vi "MB_Master Comm Tester.vi"() -> ()   [LabVIEW 2012]
doc: "Modbus Comm Tester\n\nThis VI demonstrates the usage of the Modbus Master API for both TCP and Serial connections.\nIt is also a useful tool for testing communication with your modbus device. You can test different\ncommunication parameters and coil/register address ranges without having to write any code.\n\nCopyright (c) 2016, Plasmionique Inc.\nAll rights reserved.\n\nLicense: BSD (2-Clause) - http://opensource.org/licenses/BSD-2-Clause"
uses:
  MB_Master/MB_Master.lvclass
  MB_Master_TCP/MB_Master_TCP.lvclass
  MB_ADU/MB_ADU.lvclass/MB_ADU.ctl
  MB_ADU/Read TX Data.vi
  MB_ADU/Read RX Data.vi
  MB_ADU/Read RX Timestamp.vi
  MB_Master_Serial/MB_Master_Serial.lvclass
  MB Master.lvlib
  MB_ADU/MB_ADU.lvclass
panel:
  in  "Poll Period (ms)":i32=100
  in  "Tab Control":enum32{"Page 1", "Page 2"}(tab)
  in  "Retries":i32=1
  in  "Timeout (ms)":u32=300
  in  "Flow Control":u16(ring) items=["None", "XON/XOFF", "RTS/CTS", "XON/XOFF & RTS/CTS", "DTR/DSR", "XON/XOFF & DTR/DSR"]
  in  "Parity":u16(ring) items=["None", "Odd", "Even", "Mark", "Space"]
  in  "Stop Bits":u16(ring)=10 items=["1.0"=10, "1.5"=15, "2.0"=20]
  in  "Baud Rate (bps)":u32(ring)=19200 items=["9600"=9600, "19200"=19200, "38400"=38400, "57600"=57600, "115200"=115200, "460800"=460800, "921600"=921600]
  in  "Slave Address":u8=1
  in  "Mode":enum16{"RTU", "ASCII"}(ring)
  in  "COM Port":refnum<visa-resource-name>
  in  "TCP_Port":u16=502 caption="Port"
  in  "IP Address":string="localhost"
  in  "TCP_Timeout":i32=10000 caption="Timeout (ms)"
  in  "TCP_Slave ID":u8=255 caption="Slave ID" format="%.0x"
  in  "Type":enum16{"Serial", "TCP"}(ring) caption="Connection Type"
  out "dt (ms)":u32
  in  "DI Poll":bool
  in  "IR Poll":bool
  in  "Exit":bool
  out "Last Error Time":string
  out "Last RX Time":string
  in  "Write Hld Regs":bool
  in  "Read Hld Regs":bool
  in  "HR QTY":u16=1 caption="Quantity"
  in  "HR SA":u16 caption="Starting Address" format="%.0x"
  in  "Holding Registers":u16[](array[numeric])
  in  "Read In Regs":bool
  in  "IR QTY":u16=1 caption="Quantity"
  in  "IR SA":u16 caption="Starting Address" format="%.0x"
  out "Input Registers":u16[](array[numeric])
  in  "Read DIs":bool
  in  "DI QTY":u16=1 caption="Quantity"
  in  "DI SA":u16 caption="Starting Address" format="%.0x"
  out "Discrete Inputs":bool[](array[boolean])
  in  "Write Coils":bool
  in  "Read Coils":bool
  in  "Coil QTY":u16=1 caption="Quantity"
  in  "Coil SA":u16 caption="Starting Address" format="%.0x"
  in  "Coils":bool[](array[boolean])
  out "Last TX":string
  out "Last RX":string
  out "Last Error Status":errorcluster
  out "Open?":bool
  in  "Close":bool
  in  "Open":bool
  # "Input Registers"
  # "Discrete Inputs"
  # "Communication Settngs"
  # "Communication Status"
  # "Holding Registers"
  # "Coils"
  # "See block diagram for description and usage notes."
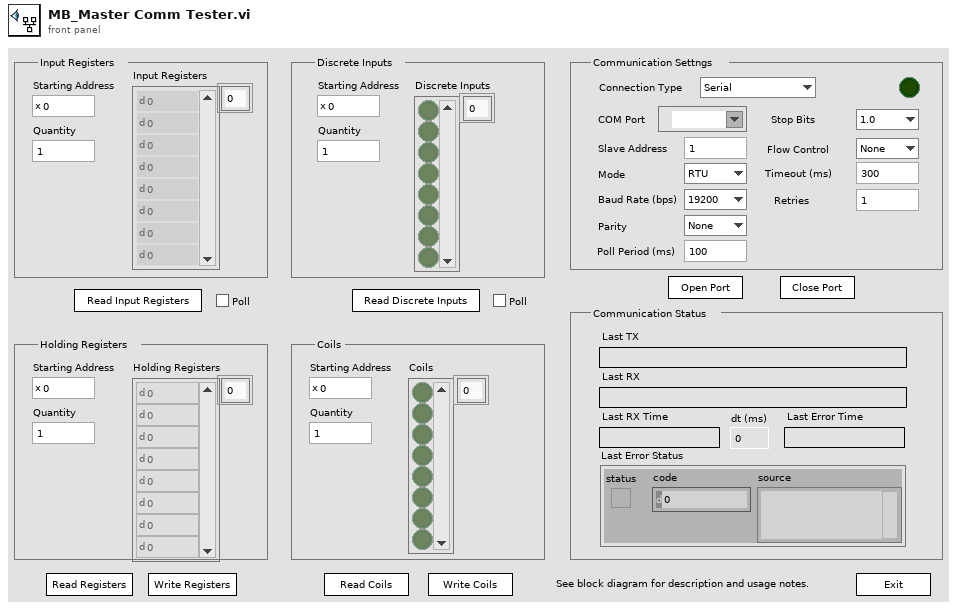
[diagram p1: front panel]
types:
  T1 = cluster{"baud rate (bps)":u32, "stop bits":u16, "parity":u16, "flow control":u16, "timeout":u32, "retries":i32}
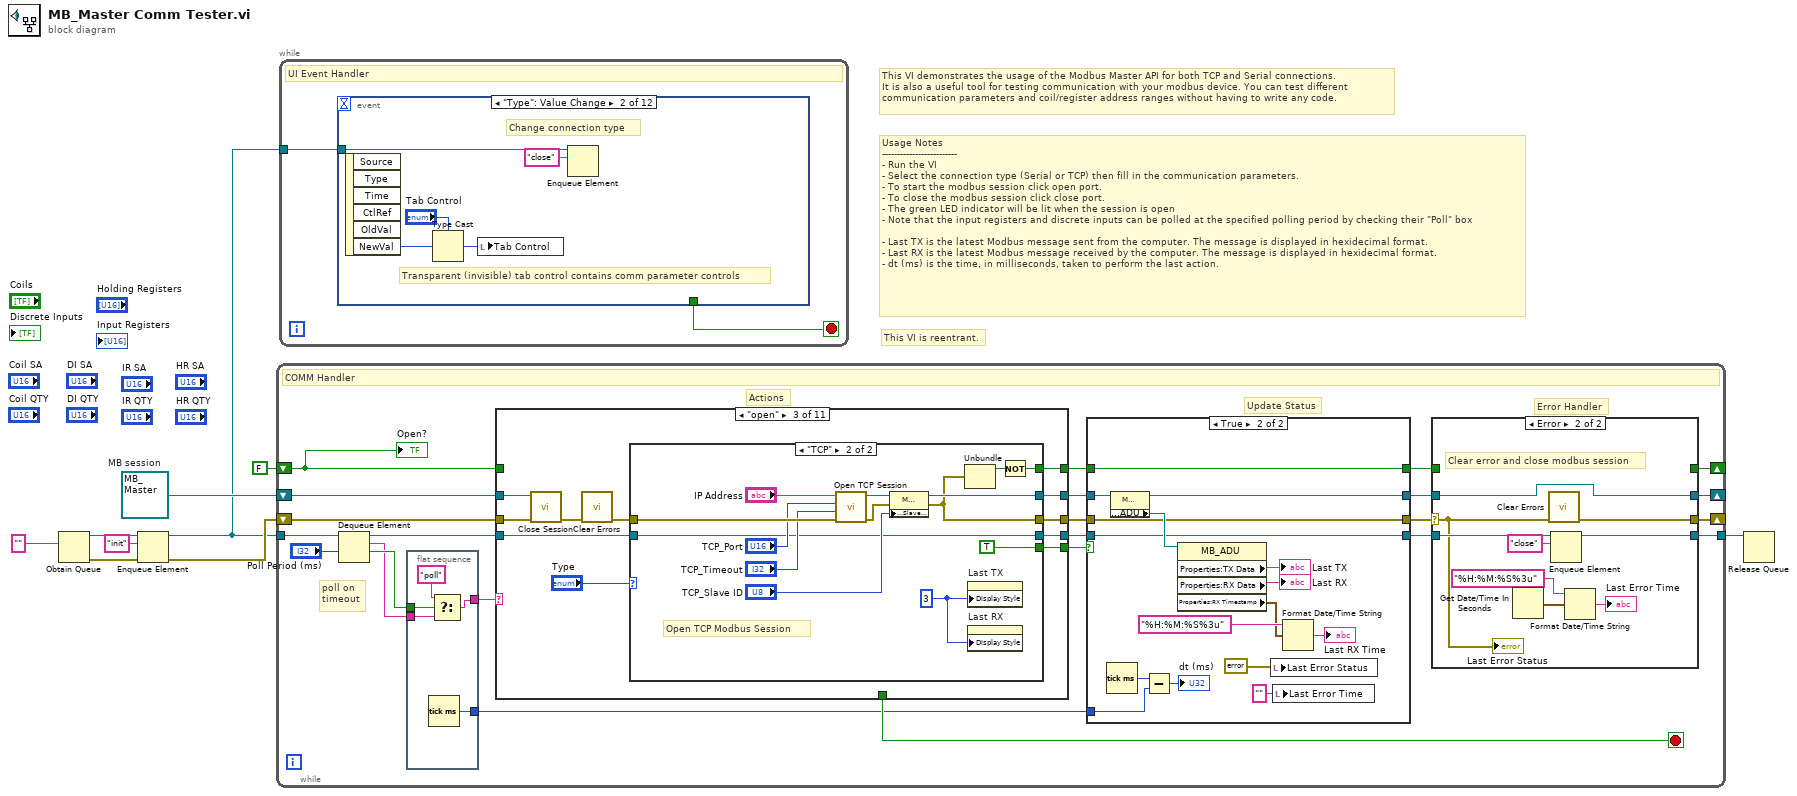
[diagram p0: block diagram]
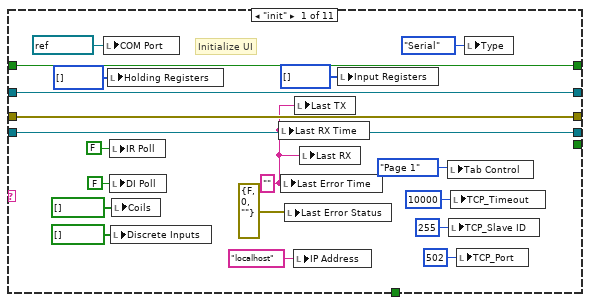
[diagram p4: hidden frame]
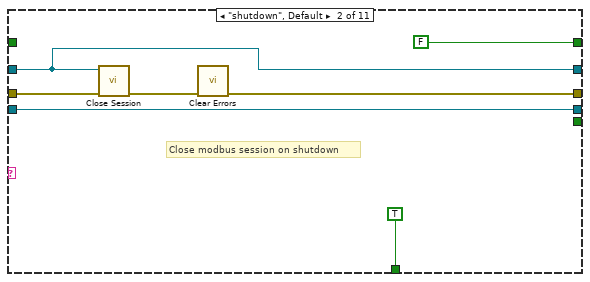
[diagram p5: hidden frame]
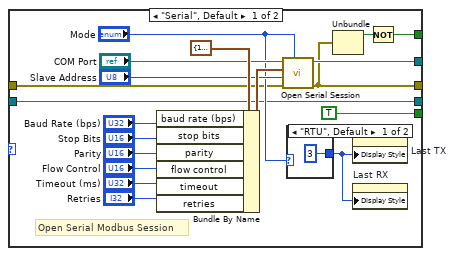
[diagram p6: hidden frame]
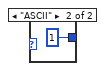
[diagram p7: hidden frame]
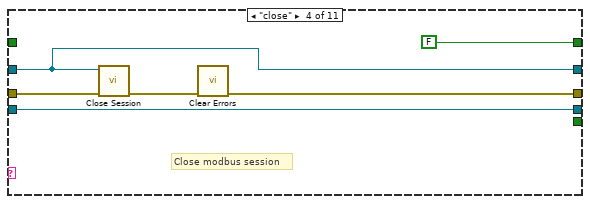
[diagram p8: hidden frame]
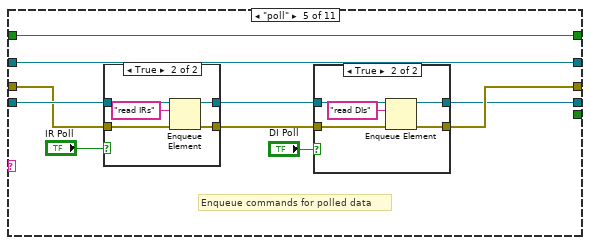
[diagram p9: hidden frame]
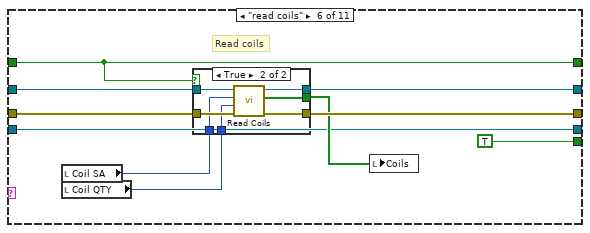
[diagram p12: hidden frame]
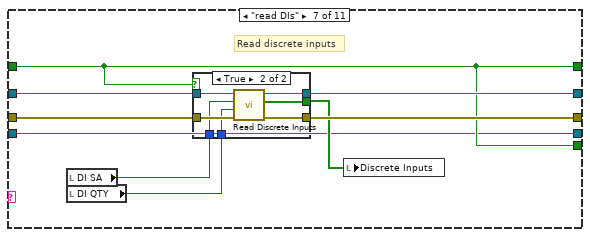
[diagram p14: hidden frame]
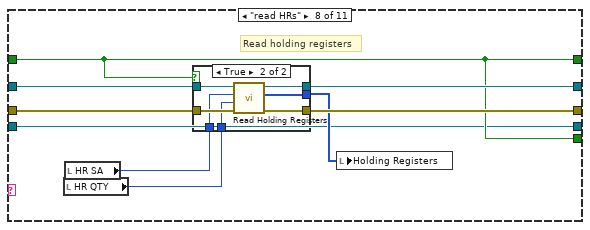
[diagram p16: hidden frame]
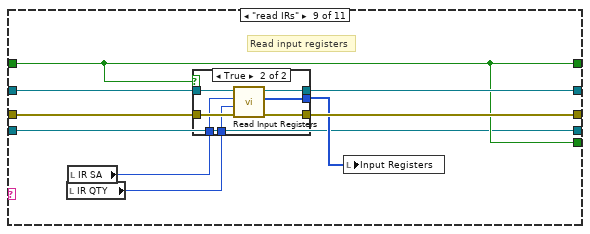
[diagram p18: hidden frame]
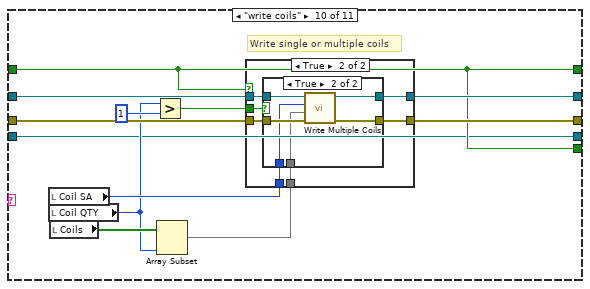
[diagram p20: hidden frame]
diagram:
  w7 = refnum<class "MB_Master.lvclass"> refnum  # MB session
  # "This VI is reentrant."
  # "Usage Notes\n-------------------------\n- Run the VI\n- Select the connection type (Serial or TCP) then fill in the communication parameters.\n- To start the modbus session click open port.\n- To close the modbus session click close port.\n- The green LED indicator will be lit when the session is open\n- Note that the input registers and discrete inputs can be polled at the specified polling period by checking their \"Poll\" box\n\n- Last TX is the latest Modbus message sent from the computer. The message is displayed in hexidecimal format.\n- Last RX is the latest Modbus message received by the computer. The message is displayed in hexidecimal format. \n- dt (ms) is the time, in milliseconds, taken to perform the last action."
  # "This VI demonstrates the usage of the Modbus Master API for both TCP and Serial connections.\nIt is also a useful tool for testing communication with your modbus device. You can test different\ncommunication parameters and coil/register address ranges without having to write any code."
  n1 = Obtain Queue(element data type="") -> (queue out=w6:refnum<queue>, error out=w4:errorcluster)  [unwired: 4 in, 1 out]
  n2 = Enqueue Element(queue=w6, element="init", error in (no error)=w4) -> (queue out=w2:refnum<queue>, error out=w3:errorcluster)  [unwired: 1 in, 1 out]
  n3 = while {
    tunnel: w2 -> [w33]
    shift-right: [w16] -> _
    shift-left: w7 -> [w32]
    shift-right: [w23] -> _
    shift-left: w3 -> [w24]
    shift-right: [w18] -> _
    shift-left: FALSE -> [w28]
    tunnel: [w22] -> w1
    stop <- w31 stop-if-true
    # "poll on\ntimeout"
    # "Actions"
    # "Error Handler"
    # "Update Status"
    # "COMM Handler"
    n4 = Dequeue Element(queue=w33, timeout in ms (-1)="Poll Period (ms)") -> (queue out=w30:refnum<queue>, element=w20:string, timed out?=w21:bool)  [unwired: 1 in, 1 out]
    n5 = flat-sequence {
      tunnel: [w51] -> w25
      tunnel: w21 -> [w50]
      tunnel: w20 -> [w49]
      tunnel: [w47] -> w19
      frame #0 {
        n6 = Tick Count (ms)() -> (millisecond timer value=w51:u32)
        n7 = Select(t="poll", s=w50, f=w49) -> (s? t:f=w47:string)
      }
    }
    n8 = case shown="\"open\"" w19 {
      tunnel: [w89 w94 w108 w146 w151 w181 w199 w217 w235 w255 w289] -> w29
      tunnel: w32 -> [w89 w94 w103 w146 w151 w183 w201 w219 w237 w258 w292]
      tunnel: [w88 w95 w107 w147 w153 w180 w198 w216 w234 w253 w287] -> w13
      tunnel: w24 -> [w88 w97 w102 w149 w156 w182 w200 w218 w236 w254 w288]
      tunnel: [_ TRUE _ _ _ _ _ _ _ _ _] -> w31
      tunnel: w30 -> [w79 w91 w99 w144 w158 w174 w193 w211 w229 w247 w281]
      tunnel: w28 -> [w86 _ _ _ w152 w178 w194 w212 w230 w248 w282]
      tunnel: [w86 FALSE w106 FALSE w152 w178 w194 w212 w230 w248 w282] -> w15
      tunnel: [_ _ w105 _ _ TRUE w194 w212 w230 w248 w282] -> w27
      tunnel: [w79 w91 w98 w144 w150 w174 w193 w211 w229 w247 w281] -> w11
      frame "init" {
        w87 = "" ("Last Error Time")
        # "Initialize UI"
        n9 = local write "COM Port"(refnum<visa-resource-name> refnum ("COM Port")) -> ()
        n10 = local write "Holding Registers"(u16[] [] ("Holding Registers")) -> ()
        n11 = local write "IR Poll"(FALSE ("IR Poll")) -> ()
        n12 = local write "DI Poll"(FALSE ("DI Poll")) -> ()
        n13 = local write "Discrete Inputs"(bool[] [] ("Coils")) -> ()
        n14 = local write "Coils"(bool[] [] ("Coils")) -> ()
        n15 = local write "Last RX Time"(w87) -> ()
        n16 = local write "Last Error Time"(w87) -> ()
        n17 = local write "Last Error Status"(errorcluster {"status"=FALSE, "code"=0, "source"=""} ("Last Error Status")) -> ()
        n18 = local write "IP Address"("localhost" ("IP Address")) -> ()
        n19 = local write "Last TX"(w87) -> ()
        n20 = local write "Last RX"(w87) -> ()
        n21 = local write "Input Registers"(u16[] [] ("Input Registers")) -> ()
        n22 = local write "Tab Control"(enum32{"Page 1", "Page 2"}."Page 1" ("Tab Control")) -> ()
        n23 = local write "TCP_Slave ID"(u8 255 ("TCP_Slave ID")) -> ()
        n24 = local write "TCP_Timeout"(10000 ("TCP_Timeout")) -> ()
        n25 = local write "TCP_Port"(u16 502 ("TCP_Port")) -> ()
        n26 = local write "Type"(enum16{"Serial", "TCP"}."Serial" ("Type")) -> ()
      }
      frame "shutdown", Default {
        # "Close modbus session on shutdown"
        n27 = call-dynamic "Close Session.vi"("error in (no error)"=w97, "MB session in"=w94) -> ("error out"=w96:errorcluster)  [unwired: 9 in]
        n28 = call <vilib>:"Clear Errors.vi"("error in (no error)"=w96) -> ("error out"=w95:errorcluster)  [unwired: 6 in]
      }
      frame "open" {
        n29 = call-dynamic "Close Session.vi"("error in (no error)"=w102, "MB session in"=w103) -> ("error out"=w104:errorcluster)  [unwired: 9 in]
        n30 = call <vilib>:"Clear Errors.vi"("error in (no error)"=w104) -> ("error out"=w101:errorcluster)  [unwired: 6 in]
        n31 = case shown="\"TCP\"" "Type" {
          tunnel: [w117 w134] -> w108
          tunnel: [w116 w132] -> w107
          tunnel: [w114 w131] -> w106
          tunnel: [TRUE TRUE] -> w105
          tunnel: w101 -> [w110 w141]
          tunnel: [w109 w135] -> w98
          tunnel: w99 -> [w109 w135]
          frame "Serial", Default {
            # "Open Serial Modbus Session"
            n32 = Bundle By Name(cluster=T1 {"baud rate (bps)"=19200, "stop bits"=10, "parity"=0, "flow control"=0, "timeout"=1000, "retries"=1} ("Serial Config"), "baud rate (bps)"="Baud Rate (bps)", "stop bits"="Stop Bits", "parity"="Parity", "flow control"="Flow Control", "timeout"="Timeout (ms)", "retries"="Retries") -> (w119:T1)
            n33 = call "Open Serial Session.vi"("Mode (RTU)"="Mode", "Error in"=w110, "Slave ID"="Slave Address", "Serial Config"=w119, "VISA Resource"="COM Port") -> ("Error out"=w116:errorcluster, "MB_Serial session"=w117:refnum<class "MB_Master_Serial.lvclass">)  [unwired: 5 in]
            n34 = case shown="\"RTU\", Default" "Mode" {
              tunnel: [u32 3 ("Display Style") u32 1 ("Display Style")] -> w111
              frame "RTU", Default {
              }
              frame "ASCII" {
              }
            }
            n35 = Unbundle(w116) -> ("status"=w115:bool)  [unwired: 2 out]
            n36 = property on="Last TX" class="Str"("Display Style"=w111) -> ()  [unwired: 2 in, 2 out]
            n37 = property on="Last RX" class="Str"("Display Style"=w111) -> ()  [unwired: 2 in, 2 out]
            n38 = Not(x=w115) -> (.not. x?=w114:bool)
          }
          frame "TCP" {
            w130 = u32 3 ("Display Style")
            # "Open TCP Modbus Session"
            n39 = call "Open TCP Session.vi"("error in (no error)"=w141, "Timeout (10000)"="TCP_Timeout", "Port (502)"="TCP_Port", "IP Address"="IP Address") -> ("error out"=w142:errorcluster, "MB_TCP session"=w143:refnum<class "MB_Master_TCP.lvclass">)  [unwired: 6 in]
            n40 = property class="MB_Master_TCP"(reference=w143, error in=w142, "Properties:Slave ID"="TCP_Slave ID") -> (reference out=w134:refnum<class "MB_Master_TCP.lvclass">, error out=w132:errorcluster)
            n41 = Unbundle(w132) -> ("status"=w133:bool)  [unwired: 2 out]
            n42 = property on="Last TX" class="Str"("Display Style"=w130) -> ()  [unwired: 2 in, 2 out]
            n43 = property on="Last RX" class="Str"("Display Style"=w130) -> ()  [unwired: 2 in, 2 out]
            n44 = Not(x=w133) -> (.not. x?=w131:bool)
          }
        }
      }
      frame "close" {
        # "Close modbus session"
        n45 = call-dynamic "Close Session.vi"("error in (no error)"=w149, "MB session in"=w146) -> ("error out"=w148:errorcluster)  [unwired: 9 in]
        n46 = call <vilib>:"Clear Errors.vi"("error in (no error)"=w148) -> ("error out"=w147:errorcluster)  [unwired: 6 in]
      }
      frame "poll" {
        # "Enqueue commands for polled data"
        n47 = case shown="True" "IR Poll" {
          tunnel: w158 -> [w168 w172]
          tunnel: [w168 w171] -> w157
          tunnel: w156 -> [w167 w170]
          tunnel: [w167 w169] -> w154
          frame False {
          }
          frame True {
            n48 = Enqueue Element(queue=w172, element="read IRs", error in (no error)=w170) -> (queue out=w171:refnum<queue>, error out=w169:errorcluster)  [unwired: 1 in, 1 out]
          }
        }
        n49 = case shown="True" "DI Poll" {
          tunnel: w157 -> [w160 w165]
          tunnel: w154 -> [w161 w164]
          tunnel: [w161 w163] -> w153
          tunnel: [w160 w162] -> w150
          frame False {
          }
          frame True {
            n50 = Enqueue Element(queue=w165, element="read DIs", error in (no error)=w164) -> (queue out=w162:refnum<queue>, error out=w163:errorcluster)  [unwired: 1 in, 1 out]
          }
        }
      }
      frame "read coils" {
        # "Read coils"
        n51 = local read "Coil SA"() -> (w177:u16)
        n52 = local read "Coil QTY"() -> (w176:u16)
        n53 = case shown="True" w178 {
          tunnel: w183 -> [w185 w192]
          tunnel: w182 -> [w184 w191]
          tunnel: [w185 w190] -> w181
          tunnel: [w184 w189] -> w180
          tunnel: w177 -> [_ w188]
          tunnel: w176 -> [_ w187]
          tunnel: [_ w186] -> w179
          frame False {
          }
          frame True {
            n54 = call "Read Coils.vi"("error in (no error)"=w191, "quantity"=w187, "starting address"=w188, "MB session in"=w192) -> ("error out"=w189:errorcluster, "Coils"=w186:bool[], "MB session out"=w190:refnum<class "MB_Master.lvclass">)  [unwired: 5 in]
          }
        }
        n55 = local write "Coils"(w179) -> ()
      }
      frame "read DIs" {
        # "Read discrete inputs"
        n56 = local read "DI SA"() -> (w196:u16)
        n57 = local read "DI QTY"() -> (w195:u16)
        n58 = case shown="True" w194 {
          tunnel: w201 -> [w203 w210]
          tunnel: w200 -> [w202 w209]
          tunnel: [w203 w208] -> w199
          tunnel: [w202 w207] -> w198
          tunnel: w196 -> [_ w206]
          tunnel: w195 -> [_ w205]
          tunnel: [_ w204] -> w197
          frame False {
          }
          frame True {
            n59 = call "Read Discrete Inputs.vi"("error in (no error)"=w209, "quantity"=w205, "starting address"=w206, "MB session in"=w210) -> ("error out"=w207:errorcluster, "Inputs"=w204:bool[], "MB session out"=w208:refnum<class "MB_Master.lvclass">)  [unwired: 5 in]
          }
        }
        n60 = local write "Discrete Inputs"(w197) -> ()
      }
      frame "read HRs" {
        # "Read holding registers"
        n61 = local read "HR QTY"() -> (w213:u16)
        n62 = local read "HR SA"() -> (w214:u16)
        n63 = case shown="True" w212 {
          tunnel: w219 -> [w221 w228]
          tunnel: w218 -> [w220 w227]
          tunnel: [w221 w226] -> w217
          tunnel: [w220 w225] -> w216
          tunnel: w214 -> [_ w224]
          tunnel: w213 -> [_ w223]
          tunnel: [_ w222] -> w215
          frame False {
          }
          frame True {
            n64 = call "Read Holding Registers.vi"("error in (no error)"=w227, "quantity"=w223, "starting address"=w224, "MB session in"=w228) -> ("error out"=w225:errorcluster, "Registers"=w222:u16[], "MB session out"=w226:refnum<class "MB_Master.lvclass">)  [unwired: 5 in]
          }
        }
        n65 = local write "Holding Registers"(w215) -> ()
      }
      frame "read IRs" {
        # "Read input registers"
        n66 = local read "IR QTY"() -> (w231:u16)
        n67 = local read "IR SA"() -> (w232:u16)
        n68 = case shown="True" w230 {
          tunnel: w237 -> [w239 w246]
          tunnel: w236 -> [w238 w245]
          tunnel: [w239 w244] -> w235
          tunnel: [w238 w243] -> w234
          tunnel: w232 -> [_ w242]
          tunnel: w231 -> [_ w241]
          tunnel: [_ w240] -> w233
          frame False {
          }
          frame True {
            n69 = call "Read Input Registers.vi"("error in (no error)"=w245, "quantity"=w241, "starting address"=w242, "MB session in"=w246) -> ("error out"=w243:errorcluster, "Registers"=w240:u16[], "MB session out"=w244:refnum<class "MB_Master.lvclass">)  [unwired: 5 in]
          }
        }
        n70 = local write "Input Registers"(w233) -> ()
      }
      frame "write coils" {
        # "Write single or multiple coils"
        n71 = local read "Coil SA"() -> (w252:u16)
        n72 = local read "Coil QTY"() -> (w250:u16)
        n73 = local read "Coils"() -> (w251:bool[])
        n74 = Greater?(x=w250, y=u16 1) -> (0:w256:bool)
        n75 = Array Subset(array=w251, length=w250) -> (w249:bool[])  [unwired: 1 in]
        n76 = case shown="True" w248 {
          tunnel: w258 -> [w260 w267]
          tunnel: w256 -> [_ w266]
          tunnel: [w260 w265] -> w255
          tunnel: w254 -> [w259 w264]
          tunnel: [w259 w263] -> w253
          tunnel: w252 -> [_ w262]
          tunnel: w249 -> [_ w261]
          frame False {
          }
          frame True {
            n77 = case shown="True" w266 {
              tunnel: w267 -> [w274 w280]
              tunnel: [w268 w279] -> w265
              tunnel: w264 -> [w273 w278]
              tunnel: [w269 w277] -> w263
              tunnel: w262 -> [w272 w276]
              tunnel: w261 -> [w271 w275]
              frame False {
                n78 = Index Array(array=w271) -> (element=w270:bool)  [unwired: 1 in]
                n79 = call "Write Single Coil.vi"("error in (no error)"=w273, "value"=w270, "address"=w272, "MB session in"=w274) -> ("error out"=w269:errorcluster, "MB session out"=w268:refnum<class "MB_Master.lvclass">)  [unwired: 6 in]
              }
              frame True {
                n80 = call "Write Multiple Coils.vi"("error in (no error)"=w278, "values"=w275, "starting address"=w276, "MB session in"=w280) -> ("error out"=w277:errorcluster, "MB session out"=w279:refnum<class "MB_Master.lvclass">)  [unwired: 6 in]
              }
            }
          }
        }
      }
      frame "write HRs" {
        # "Write single or multiple holding registers"
        n81 = local read "Holding Registers"() -> (w285:u16[])
        n82 = local read "HR QTY"() -> (w284:u16)
        n83 = local read "HR SA"() -> (w286:u16)
        n84 = Greater?(x=w284, y=u16 1) -> (0:w290:bool)
        n85 = Array Subset(array=w285, length=w284) -> (w283:u16[])  [unwired: 1 in]
        n86 = case shown="True" w282 {
          tunnel: w292 -> [w294 w301]
          tunnel: w290 -> [_ w300]
          tunnel: [w294 w299] -> w289
          tunnel: w288 -> [w293 w298]
          tunnel: [w293 w297] -> w287
          tunnel: w286 -> [_ w296]
          tunnel: w283 -> [_ w295]
          frame False {
          }
          frame True {
            n87 = case shown="True" w300 {
              tunnel: w301 -> [w308 w314]
              tunnel: [w302 w313] -> w299
              tunnel: w298 -> [w307 w312]
              tunnel: [w303 w311] -> w297
              tunnel: w296 -> [w306 w310]
              tunnel: w295 -> [w305 w309]
              frame False {
                n88 = Index Array(array=w305) -> (element=w304:u16)  [unwired: 1 in]
                n89 = call "Write Single Register.vi"("error in (no error)"=w307, "value"=w304, "address"=w306, "MB session in"=w308) -> ("error out"=w303:errorcluster, "MB session out"=w302:refnum<class "MB_Master.lvclass">)  [unwired: 6 in]
              }
              frame True {
                n90 = call "Write Multiple Registers.vi"("error in (no error)"=w312, "values"=w309, "starting address"=w310, "MB session in"=w314) -> ("error out"=w311:errorcluster, "MB session out"=w313:refnum<class "MB_Master.lvclass">)  [unwired: 6 in]
              }
            }
          }
        }
      }
    }
    n91 = case shown="True" w27 {
      tunnel: w29 -> [w55 w56]
      tunnel: [w55 w69] -> w17
      tunnel: w25 -> [_ w63]
      tunnel: w15 -> [w54 w59]
      tunnel: [w54 w59] -> w14
      tunnel: w13 -> [w53 w58]
      tunnel: [w53 w58] -> w12
      tunnel: w11 -> [w52 w57]
      tunnel: [w52 w57] -> w10
      frame False {
      }
      frame True {
        n92 = Tick Count (ms)() -> (millisecond timer value=w62:u32)
        n93 = property class="MB_Master"(reference=w56) -> (reference out=w69:refnum<class "MB_Master.lvclass">, "Properties:ADU"=w70:refnum<class "MB_ADU.lvclass">)  [unwired: 1 in, 1 out]
        n94 = Subtract(x=w62, y=w63) -> (x-y=→"dt (ms)":u32)
        n95 = property class="MB_ADU"(reference=w70) -> ("Properties:TX Data"=→"Last TX":string, "Properties:RX Data"=→"Last RX":string, "Properties:RX Timestamp"=w60:timestamp)  [unwired: 1 in, 2 out]
        n96 = local write "Last Error Status"(errorcluster {"status"=FALSE, "code"=0, "source"=""} ("Last Error Status")) -> ()
        n97 = local write "Last Error Time"("" ("Last Error Time")) -> ()
        n98 = Format Date/Time String(time format string (%c)="%H:%M:%S%3u", seconds (now)=w60) -> (date/time string=→"Last RX Time":string)  [unwired: 1 in]
      }
    }
    n99 = case shown="Error" w12 {
      selector: w12 -> [w37 w39]
      tunnel: [w37 w43] -> w23
      tunnel: w10 -> [w36 w41]
      tunnel: [w36 w40] -> w22
      tunnel: w14 -> [w35 _]
      tunnel: [w35 _] -> w18
      tunnel: w17 -> [w34 w38]
      tunnel: [w34 w38] -> w16
      frame No Error {
      }
      frame Error {
        # "Clear error and close modbus session"
        n100 = Get Date/Time In Seconds() -> (seconds since 1Jan1904=w44:timestamp)
        n101 = call <vilib>:"Clear Errors.vi"("error in (no error)"=w39) -> ("error out"=w43:errorcluster)  [unwired: 6 in]
        n102 = Enqueue Element(queue=w41, element="close") -> (queue out=w40:refnum<queue>)  [unwired: 2 in, 2 out]
        n103 = Format Date/Time String(time format string (%c)="%H:%M:%S%3u", seconds (now)=w44) -> (date/time string=→"Last Error Time":string)  [unwired: 1 in]
        "Last Error Status" <- w39
      }
    }
    "Open?" <- w28
  }
  n104 = while {
    tunnel: w2 -> [w316]
    stop <- w315 stop-if-true
    # "UI Event Handler"
    n105 = event shown="[1] \"Type\": Value Change" {
      selector: _ -> [_ _ _ _ _ _ _ _ _ _ _ _]
      dyn-events: _ -> [_ _ _ _ _ _ _ _ _ _ _ _]
      timeout: _ -> [_ _ _ _ _ _ _ _ _ _ _ _]
      tunnel: w316 -> [_ w320 w323 w324 w326 w328 w330 w332 w334 w336 w338 w342]
      tunnel: [_ _ _ _ _ _ _ _ _ _ TRUE TRUE] -> w315
      event Timeout {
        n106 = event-data() -> ()  [unwired: 1 in, 3 out]
      }
      event "Type": Value Change {
        # "Transparent (invisible) tab control contains comm parameter controls"
        # "Change connection type"
        n107 = event-data() -> ("NewVal"=w319:enum16{"Serial", "TCP"})  [unwired: 1 in, 5 out]
        n108 = Type Cast(type="Tab Control", x=w319) -> (*(type *) &x=w317:enum32{"Page 1", "Page 2"})
        n109 = local write "Tab Control"(w317) -> ()
        n110 = Enqueue Element(queue=w320, element="close") -> ()  [unwired: 2 in, 3 out]
      }
      event "Open": Value Change {
        # "Open modbus session"
        n111 = event-data() -> ()  [unwired: 1 in, 6 out]
        n112 = Enqueue Element(queue=w323, element="open") -> ()  [unwired: 2 in, 3 out]
      }
      event "Close": Value Change {
        # "Close modbus session"
        n113 = event-data() -> ()  [unwired: 1 in, 6 out]
        n114 = Enqueue Element(queue=w324, element="close") -> ()  [unwired: 2 in, 3 out]
      }
      event "Read Coils": Value Change {
        n115 = event-data() -> ()  [unwired: 1 in, 6 out]
        n116 = Enqueue Element(queue=w326, element="read coils") -> ()  [unwired: 2 in, 3 out]
      }
      event "Read DIs": Value Change {
        n117 = event-data() -> ()  [unwired: 1 in, 6 out]
        n118 = Enqueue Element(queue=w328, element="read DIs") -> ()  [unwired: 2 in, 3 out]
      }
      event "Write Coils": Value Change {
        n119 = event-data() -> ()  [unwired: 1 in, 6 out]
        n120 = Enqueue Element(queue=w330, element="write coils") -> ()  [unwired: 2 in, 3 out]
      }
      event "Read In Regs": Value Change {
        n121 = event-data() -> ()  [unwired: 1 in, 6 out]
        n122 = Enqueue Element(queue=w332, element="read IRs") -> ()  [unwired: 2 in, 3 out]
      }
      event "Read Hld Regs": Value Change {
        n123 = event-data() -> ()  [unwired: 1 in, 6 out]
        n124 = Enqueue Element(queue=w334, element="read HRs") -> ()  [unwired: 2 in, 3 out]
      }
      event "Write Hld Regs": Value Change {
        n125 = event-data() -> ()  [unwired: 1 in, 6 out]
        n126 = Enqueue Element(queue=w336, element="write HRs") -> ()  [unwired: 2 in, 3 out]
      }
      event Panel Close? {
        n127 = event-data() -> ()  [unwired: 1 in, 4 out]
        n128 = Enqueue Element(queue=w338, element="shutdown") -> ()  [unwired: 2 in, 3 out]
        n129 = event-data("Discard?"=TRUE) -> ()  [unwired: 1 in, 1 out]
      }
      event "Exit": Value Change {
        n130 = event-data() -> ()  [unwired: 1 in, 6 out]
        n131 = Enqueue Element(queue=w342, element="shutdown") -> ()  [unwired: 2 in, 3 out]
      }
    }
  }
  n132 = Release Queue(queue=w1) -> ()  [unwired: 2 in, 3 out]
